vi "Finding Index.vi"(10 "Search Setting":T1, 11 "Array to be Tested":dbl[](array[numeric])) -> (3 "Indexis taht falls in the range":dbl[](array[numeric]))   [LabVIEW 2017]
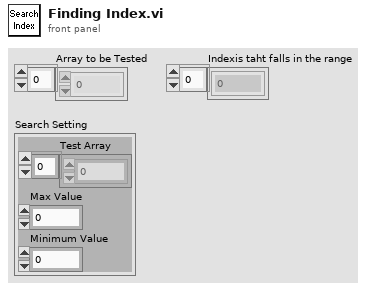
[diagram p1: front panel]
types:
  T1 = cluster{"Test Array":dbl[], "Max Value":dbl, "Minimum Value":dbl}
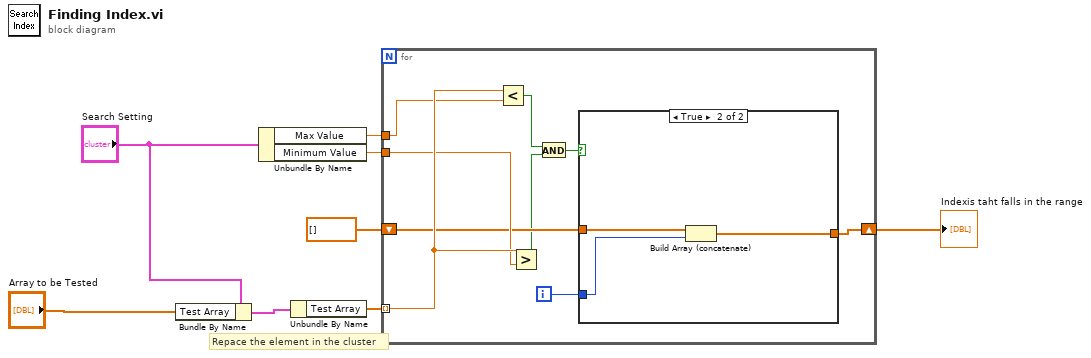
[diagram p0: block diagram]
diagram:
  # "Repace the element in the cluster"
  n1 = Bundle By Name(cluster="Search Setting", "Test Array"="Array to be Tested") -> (w1:T1)
  n2 = Unbundle By Name("Search Setting") -> ("Max Value"=w4:dbl, "Minimum Value"=w5:dbl)
  n3 = Unbundle By Name(w1) -> ("Test Array"=w3:dbl[])
  n4 = for {
    tunnel: w3 -> [w17] mode=indexing
    tunnel: w4 -> [w16]
    tunnel: w5 -> [w15]
    shift-right: [w12] -> w7
    shift-left: dbl[] [] -> [w14]
    i -> [w13]
    n5 = Less?(x=w17, y=w16) -> (x < y?=w11:bool)
    n6 = Greater?(x=w17, y=w15) -> (0:w10:bool)
    n7 = And(x=w11, y=w10) -> (x .and. y?=w9:bool)
    n8 = case shown="True" w9 {
      tunnel: w14 -> [w18 w21]
      tunnel: w13 -> [_ w20]
      tunnel: [w18 w19] -> w12
      frame False {
      }
      frame True {
        n9 = Build Array (concatenate)(w21, w20) -> (w19:dbl[])
      }
    }
  }
  "Indexis taht falls in the range" <- w7
